vi "TrayIcon.vi"(7 "Mouseover Text":string, 10 "error in (no error)":errorcluster, 11 "Icon Path":path) -> (2 "error out":errorcluster, 3 "NotifyIcon out":refnum<class "MGI_TrayIcon.lvclass">)   [LabVIEW 2016, in "MGI_TrayIcon.lvclass"]
doc: "This will create a new tray icon with the right click menu as defined. When the item is double clicked on it will automatically click the TrayItem specified as default item.\n\nThis menu type requires the .NET framework, therefore will only work on windows.\n\nAuthored by Derek E. Trepanier\nsupport@mooregoodideas.com\nwww.mooregoodideas.com\n\nCopyright (c) 2012, Moore Good Ideas, Inc.\n\nAll rights reserved.\n\nRedistribution and use in source and binary forms, with or without modification, are permitted provided that the following conditions are met:\n\n * Redistributions of source code must retain the above copyright notice, this list of conditions and the following disclaimer.\n * Redistributions in binary form must reproduce the above copyright notice, this list of conditions and the following disclaimer in the documentation and/or other materials provided with the distribution.\n * Neither the name of Moore Good Ideas, Inc. nor the names of its contributors may be used to endorse or promote products derived from this software without specific prior written permission.\n\nTHIS SOFTWARE IS PROVIDED BY THE COPYRIGHT HOLDERS AND CONTRIBUTORS \"AS IS\" AND ANY EXPRESS OR IMPLIED WARRANTIES, INCLUDING, BUT NOT LIMITED TO, THE IMPLIED WARRANTIES OF MERCHANTABILITY AND FITNESS FOR A PARTICULAR PURPOSE ARE DISCLAIMED. IN NO EVENT SHALL THE COPYRIGHT OWNER OR CONTRIBUTORS BE LIABLE FOR ANY DIRECT, INDIRECT, INCIDENTAL, SPECIAL, EXEMPLARY, OR CONSEQUENTIAL DAMAGES (INCLUDING, BUT NOT LIMITED TO, PROCUREMENT OF SUBSTITUTE GOODS OR SERVICES; LOSS OF USE, DATA, OR PROFITS; OR BUSINESS INTERRUPTION) HOWEVER CAUSED AND ON ANY THEORY OF LIABILITY, WHETHER IN CONTRACT, STRICT LIABILITY, OR TORT (INCLUDING NEGLIGENCE OR OTHERWISE) ARISING IN ANY WAY OUT OF THE USE OF THIS SOFTWARE, EVEN IF ADVISED OF THE POSSIBILITY OF SUCH DAMAGE."
uses:
  <userlib>/_MGI/Menu Building/MenuTypes/TrayIcon/MGI_TrayIcon.lvclass
  <userlib>/_MGI/Menu Building/MenuTypes/TrayIcon/MGI_TrayIcon.lvclass/MGI_TrayIcon.ctl
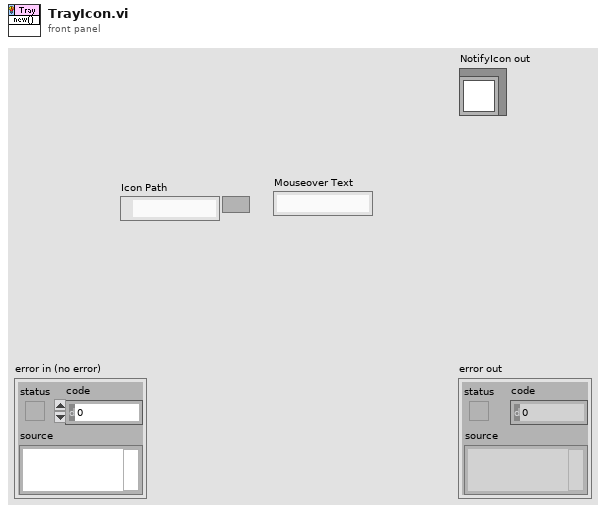
[diagram p1: front panel]
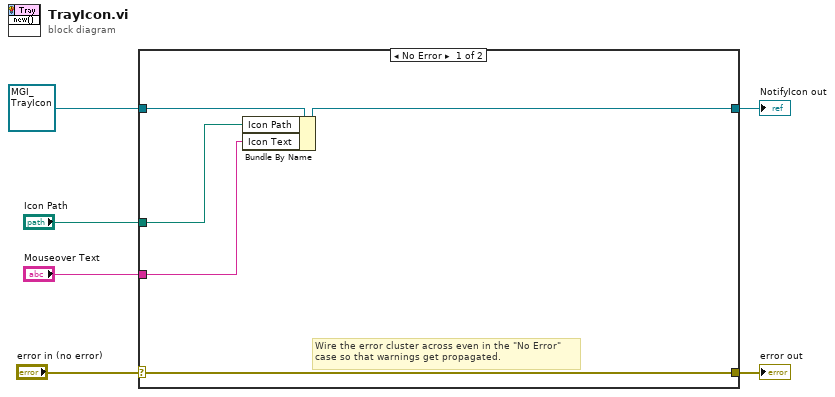
[diagram p0: block diagram]
diagram:
  n1 = case shown="No Error" "error in (no error)" {
    selector: "error in (no error)" -> [w10 w13]
    tunnel: [w10 w13] -> w5
    tunnel: [w9 w12] -> w3
    tunnel: refnum<class "MGI_TrayIcon.lvclass"> refnum ("NotifyIcon in") -> [w11 w12]
    tunnel: "Icon Path" -> [w8 _]
    tunnel: "Mouseover Text" -> [w7 _]
    frame No Error {
      # "Wire the error cluster across even in the \"No Error\"\ncase so that warnings get propagated."
      n2 = Bundle By Name(cluster=w11, "Icon Path"=w8, "Icon Text"=w7) -> (w9:refnum<class "MGI_TrayIcon.lvclass">)
    }
    frame Error {
    }
  }
  "error out" <- w5
  "NotifyIcon out" <- w3
